vi "LASERs_ Crl_AE.vi"(7 "Action":enum16{"READ", "WRITE"}(ring), 10 "Detectors Parameters In":T1 {"STED Power (V)" scale=0.0..10.0}) -> (2 "Detectors Parameters Out":T1 {"STED Power (V)" scale=0.0..10.0})   [LabVIEW 2014]
uses:
  Host VIs/Laser Controls.ctl
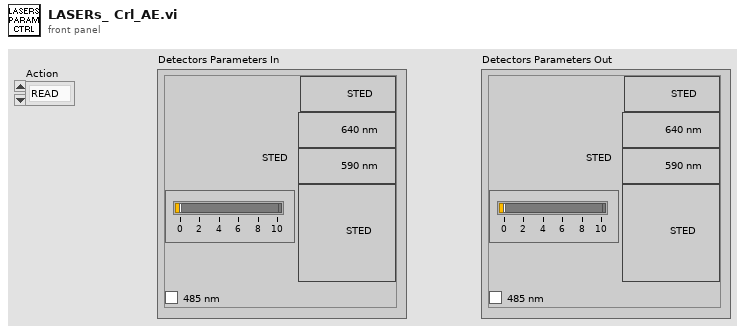
[diagram p1: front panel]
types:
  T1 = typedef "Laser Controls.ctl" = cluster{"STED Power (V)":dbl, "STED":bool, "650 nm":bool, "590 nm":bool, "485 nm":bool, "Manual Control":bool}
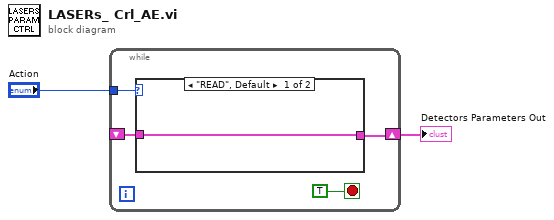
[diagram p0: block diagram]
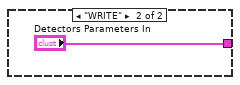
[diagram p2: hidden frame]
diagram:
  n1 = while {
    tunnel: "Action" -> [w5]
    shift-right: [w4] -> w1
    shift-left: _ -> [w3]
    stop <- TRUE stop-if-true
    n2 = case shown="\"READ\", Default" w5 {
      tunnel: [w7 "Detectors Parameters In"] -> w4
      tunnel: w3 -> [w7 _]
      frame "READ", Default {
      }
      frame "WRITE" {
      }
    }
  }
  "Detectors Parameters Out" <- w1
